vi "Serialize.vi"(8 "error in (no error)":errorcluster, 11 "VIPC Apply in":refnum<class "VIPC Apply.lvclass">) -> (0 "error out":errorcluster, 2 "Text":string)   [LabVIEW 2014, in "VIPC Apply.lvclass"]
uses:
  VIPC Apply.lvclass
  Shared/Controls/VIPC Apply - STYP.ctl
  VIPC Apply.lvclass/VIPC Apply.ctl
  Read LV Version.vi
  Read VIPC_Path.vi
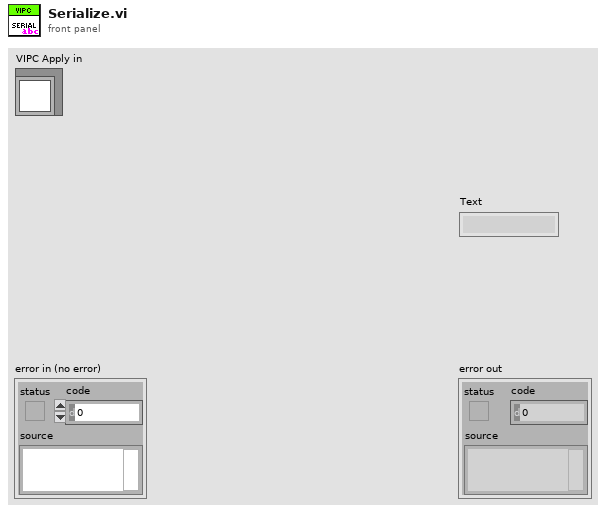
[diagram p1: front panel]
types:
  T1 = typedef "VIPC Apply - STYP.ctl" = cluster{"VIPC Path":string, "LabVIEW Version":string}
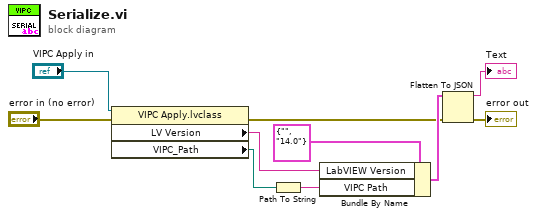
[diagram p0: block diagram]
diagram:
  n1 = property class="VIPC Apply.lvclass"(reference="VIPC Apply in", error in="error in (no error)") -> (error out=w4:errorcluster, "LV Version"=w8:string, "VIPC_Path"=w7:path)  [unwired: 1 out]
  n2 = Path To String(path=w7) -> (string=w6:string)
  n3 = Bundle By Name(cluster=T1 {"VIPC Path"="", "LabVIEW Version"="14.0"} ("VIPB Build"), "LabVIEW Version"=w8, "VIPC Path"=w6) -> (w5:T1)
  n4 = Flatten To JSON(anything=w5, error in (no error)=w4) -> (JSON string=→"Text":string, 11:→"error out":errorcluster)  [unwired: 1 in]
